vi "Read Given Name.vi"(11 "UniqueName in":refnum<class "UniqueName.lvclass">) -> (2 "Given Name":string, 3 "UniqueName out":refnum<class "UniqueName.lvclass">)   [LabVIEW 2013, in "UniqueName.lvlib" / "UniqueName.lvclass"]
uses:
  UniqueName.lvclass
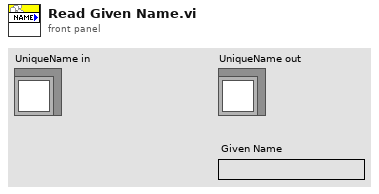
[diagram p1: front panel]
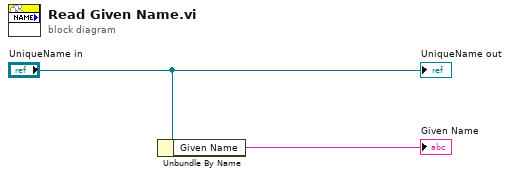
[diagram p0: block diagram]
diagram:
  n1 = Unbundle By Name("UniqueName in") -> ("Given Name"=→"Given Name":string)
  "UniqueName out" <- "UniqueName in"
